vi "count-tsk2.vi"() -> ()   [LabVIEW 2020]
panel:
  in  "reset":bool
  out "count":dbl
  in  "stop":bool
  in  "count down":bool
  in  "count up":bool
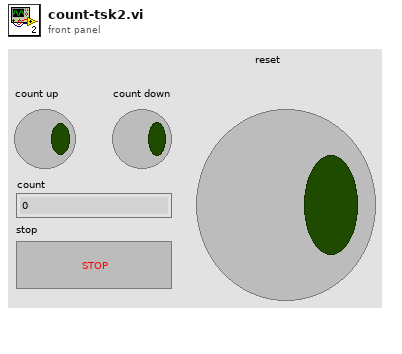
[diagram p1: front panel]
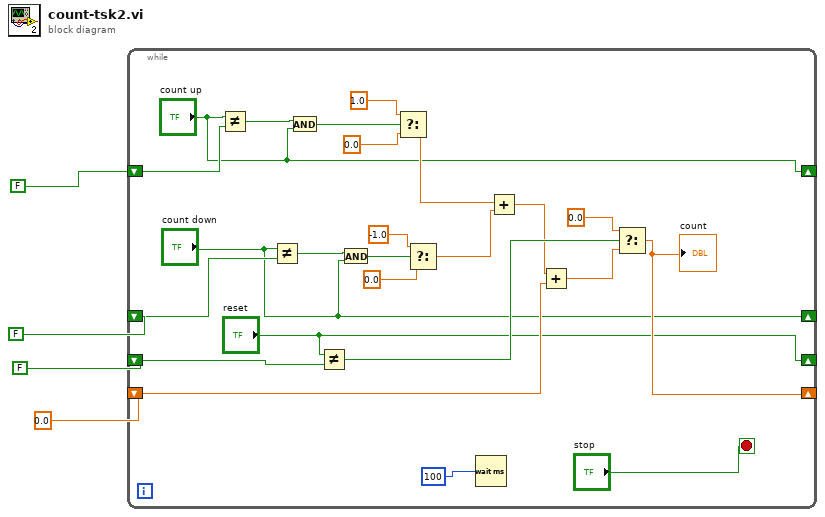
[diagram p0: block diagram]
diagram:
  n1 = while {
    shift-right: [w10] -> _
    shift-left: 0.0 -> [w12]
    shift-right: ["count down"] -> _
    shift-left: FALSE -> [w21]
    shift-right: ["count up"] -> _
    shift-left: FALSE -> [w26]
    shift-right: ["reset"] -> _
    shift-left: FALSE -> [w15]
    stop <- "stop" stop-if-true
    n2 = Not Equal?(x="count up", y=w26) -> (x != y?=w27:bool)
    n3 = Not Equal?(x="count down", y=w21) -> (x != y?=w22:bool)
    n4 = And(x=w27, y="count up") -> (x .and. y?=w25:bool)
    n5 = Not Equal?(x="reset", y=w15) -> (x != y?=w14:bool)
    n6 = And(x=w22, y="count down") -> (x .and. y?=w20:bool)
    n7 = Select(t=1.0, s=w25, f=0.0) -> (s? t:f=w17:dbl)
    n8 = Select(t=-1.0, s=w20, f=0.0) -> (s? t:f=w16:dbl)
    n9 = Wait (ms)(milliseconds to wait=100) -> ()  [unwired: 1 out]
    n10 = Add(x=w17, y=w16) -> (x+y=w13:dbl)
    n11 = Add(x=w13, y=w12) -> (x+y=w11:dbl)
    n12 = Select(t=0.0, s=w14, f=w11) -> (s? t:f=w10:dbl)
    "count" <- w10
  }
